vi "Lab2.vi"() -> ()   [LabVIEW 2019]
panel:
  in  "stop":bool
  out "Boolean":bool
  in  "Button":bool
  out "Green":bool
  out "Yellow":bool
  out "Red":bool
  out "Walk":bool
  out "Don't_Walk":bool
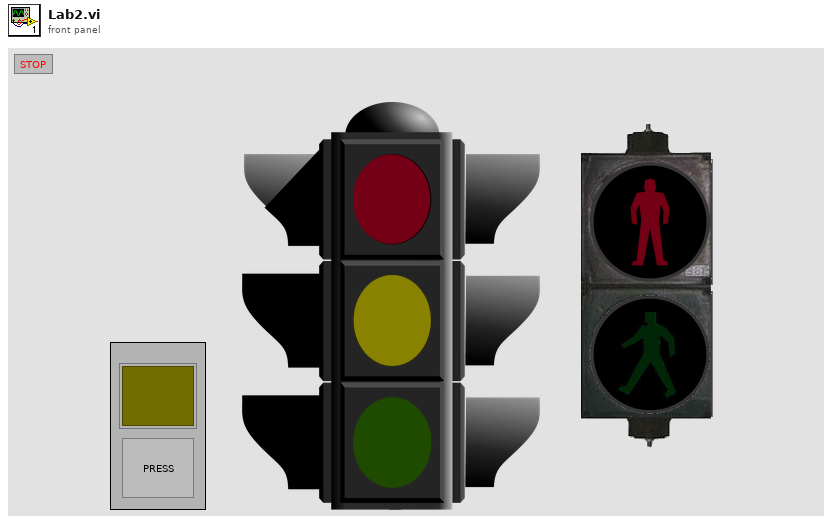
[diagram p1: front panel]
types:
  T1 = enum16{"Green", "Yellow", "PedestrianYellow", "Red", "PedestrianGreen", "PedestrianBlinking"}
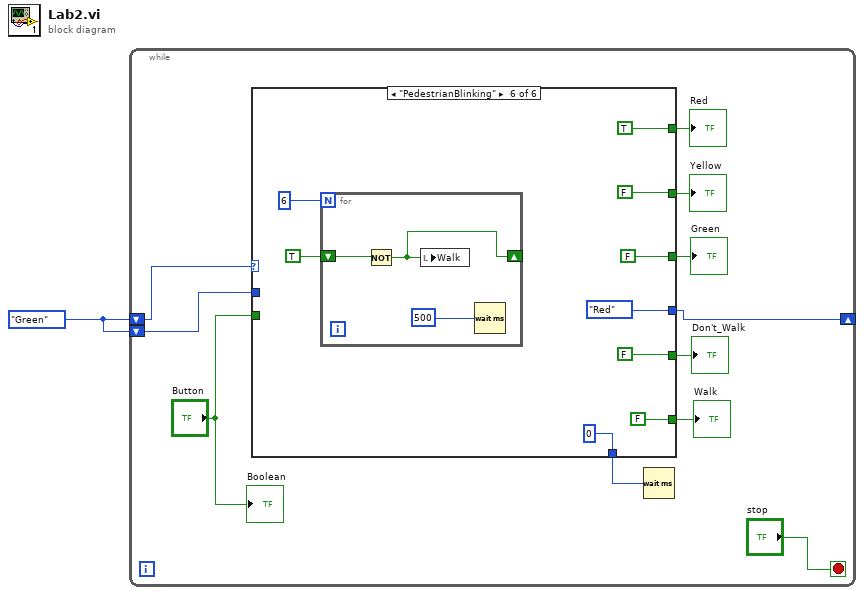
[diagram p0: block diagram]
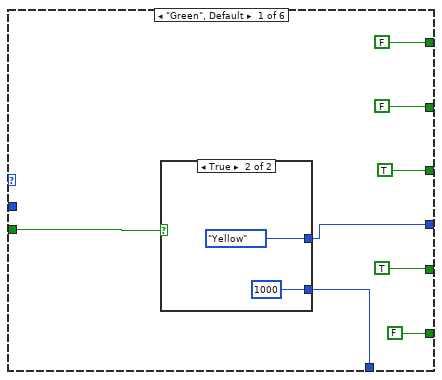
[diagram p2: hidden frame]
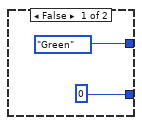
[diagram p3: hidden frame]
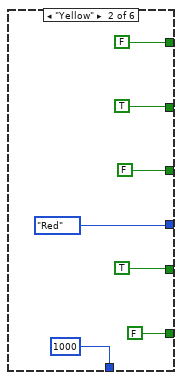
[diagram p4: hidden frame]
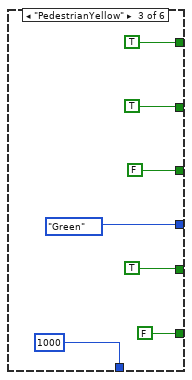
[diagram p5: hidden frame]
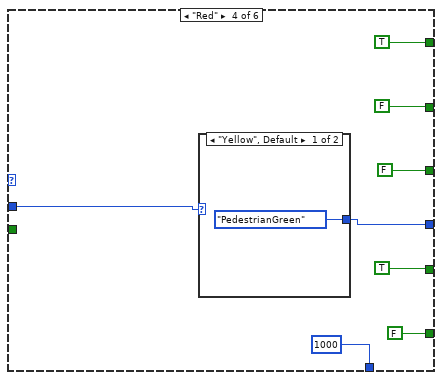
[diagram p6: hidden frame]
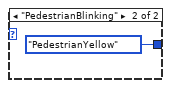
[diagram p7: hidden frame]
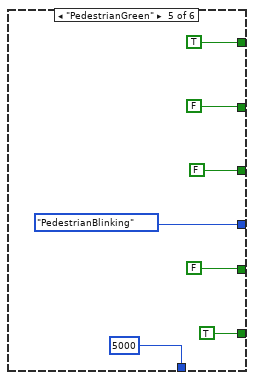
[diagram p8: hidden frame]
diagram:
  w1 = T1."Green"
  n1 = while {
    shift-right: [w3] -> _
    shift-left: w1 -> [w11]
    shift-left: w1 -> [w2]
    stop <- "stop" stop-if-true
    n2 = case shown="\"PedestrianBlinking\"" w11 {
      tunnel: [FALSE FALSE TRUE TRUE TRUE TRUE] -> w10
      tunnel: [FALSE TRUE TRUE FALSE FALSE FALSE] -> w9
      tunnel: [TRUE FALSE FALSE FALSE FALSE FALSE] -> w8
      tunnel: [TRUE TRUE TRUE TRUE FALSE FALSE] -> w7
      tunnel: [FALSE FALSE FALSE FALSE TRUE FALSE] -> w6
      tunnel: [w13 1000 1000 1000 5000 0] -> w5
      tunnel: "Button" -> [w15 _ _ _ _ _]
      tunnel: [w14 T1."Red" T1."Green" w39 T1."PedestrianBlinking" T1."Red"] -> w3
      tunnel: w2 -> [_ _ _ w40 _ _]
      frame "Green", Default {
        n3 = case shown="True" w15 {
          tunnel: [T1."Green" T1."Yellow"] -> w14
          tunnel: [0 1000] -> w13
          frame False {
          }
          frame True {
          }
        }
      }
      frame "Yellow" {
      }
      frame "PedestrianYellow" {
      }
      frame "Red" {
        n4 = case shown="\"Yellow\", Default" w40 {
          tunnel: [T1."PedestrianGreen" T1."PedestrianYellow"] -> w39
          frame "Yellow", Default {
          }
          frame "PedestrianBlinking" {
          }
        }
      }
      frame "PedestrianGreen" {
      }
      frame "PedestrianBlinking" {
        n5 = for {
          N: 6 -> [_]
          shift-right: [w66] -> _
          shift-left: TRUE -> [w67]
          n6 = Not(x=w67) -> (.not. x?=w66:bool)
          n7 = local write "Walk"(w66) -> ()
          n8 = Wait (ms)(milliseconds to wait=500) -> ()  [unwired: 1 out]
        }
      }
    }
    "Don't_Walk" <- w7
    "Walk" <- w6
    "Red" <- w10
    "Yellow" <- w9
    "Green" <- w8
    n9 = Wait (ms)(milliseconds to wait=w5) -> ()  [unwired: 1 out]
    "Boolean" <- "Button"
  }
